vi "Voice_Freq_Amp_Check.vi"(8 "error in (no error)":errorcluster, 11 "IN":T1={"step name 1"="", "updata 2"="750~0.22", "limitdata 3"="650~0.101", "load vi name 4"="", "parameter 5"=""}) -> (0 "error out":errorcluster, 3 "Cluster":T2)   [LabVIEW 2013]
uses:
  <vilib>/sound2/lvsound2.llb/Sampling Mode.ctl
  <vilib>/sound2/lvsound2.llb/Sound Data Format.ctl
  <vilib>/sound2/lvsound2.llb/Sound Input Read (DBL).vi
  <vilib>/measure/matone.llb/Extract Single Tone Information N Chan.vi
  <vilib>/measure/NI_MAPro.lvlib
panel:
  out "array":string[](array[string])
  out "Array":bool[](array[boolean])
  out "number":i32
  # "Hi: 750~0.22"
  # "Lo: 650~0.101"
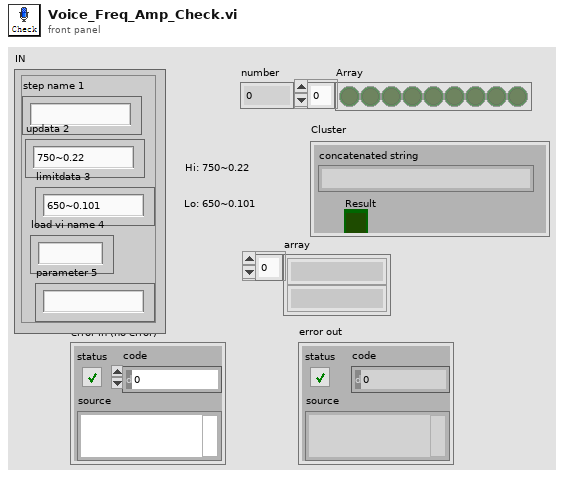
[diagram p1: front panel]
types:
  T1 = cluster{"step name 1":string, "updata 2":string, "limitdata 3":string, "load vi name 4":string, "parameter 5":string}
  T2 = cluster{"concatenated string":string, "Result":bool}
  T3 = typedef "Sound Data Format.ctl" = cluster{"sample rate (S/s)":dbl, "number of channels":i32, "bits per sample":i32}
  T4 = typedef "Sampling Mode.ctl" = i32
  T5 = typedef "Sound Input Task ID.ctl" = u32
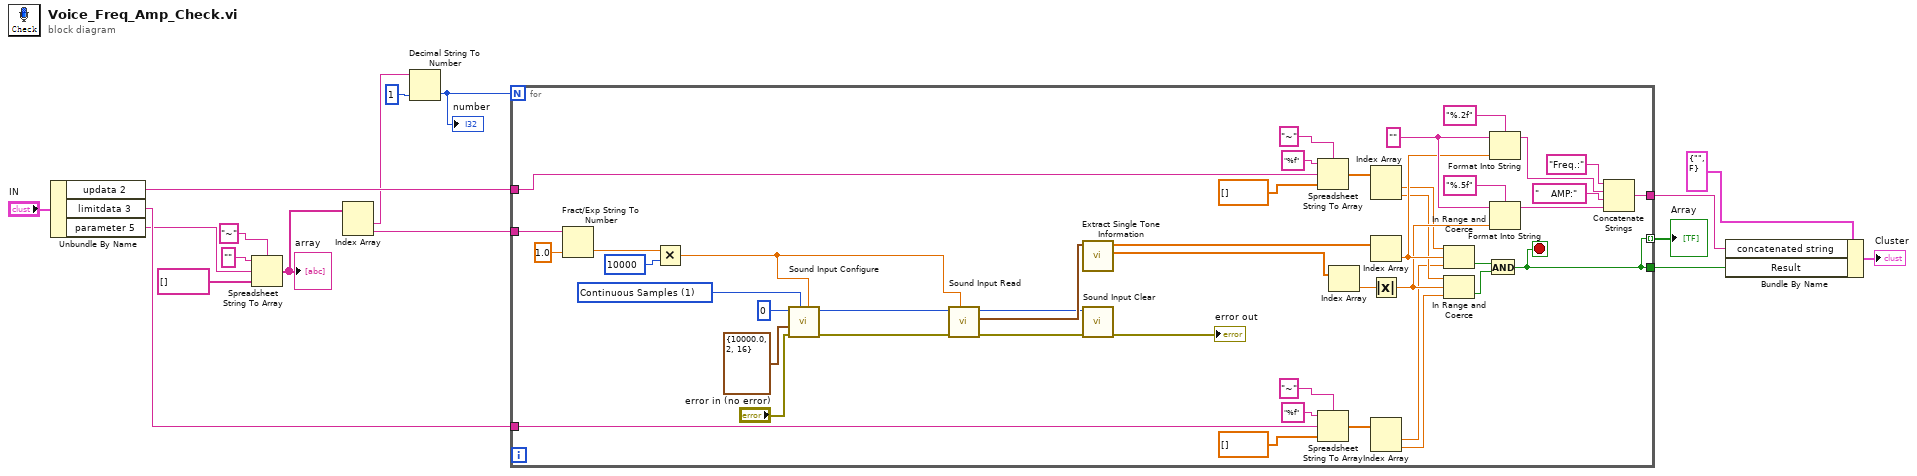
[diagram p0: block diagram]
diagram:
  n1 = Unbundle By Name("IN") -> ("updata 2"=w12:string, "limitdata 3"=w11:string, "parameter 5"=w7:string)
  n2 = Spreadsheet String To Array(delimiter (Tab)="~", format string="", spreadsheet string=w7, array type (2D Dbl)=string[] []) -> (array=w3:string[])
  "array" <- w3
  n3 = Index Array(array=w3) -> (element #1=w2:string, element #2=w1:string)  [unwired: 2 in]
  n4 = Decimal String To Number(string=w2, default (0L)=1 ("default (0 I32)")) -> (number=w9:i32)  [unwired: 1 in, 1 out]
  "number" <- w9
  n5 = for {
    N: w9 -> [_]
    tunnel: [w38] -> w15
    tunnel: [w23] -> w14
    tunnel: w12 -> [w25]
    tunnel: w11 -> [w24]
    tunnel: [w23] -> w8 mode=indexing
    tunnel: w1 -> [w22]
    stop <- w23 stop-if-true
    w49 = "" ("initial string")
    w57 = T4 1 items=["Finite Samples", "Continuous Samples"] ("sample mode")
    n6 = Fract/Exp String To Number(string=w22, default (0 dbl)=1.0 ("default (0 DBL)")) -> (number=w20:dbl)  [unwired: 2 in, 1 out]
    n7 = Multiply(x=w20, y=10000 ("Number of Samples/ch")) -> (x*y=w19:dbl)
    n8 = call <vilib>:"Sound Input Configure.vi"("number of samples/ch"=w19, "sample mode"=w57, "error in (no error)"="error in (no error)", "sound format"=T3 {"sample rate (S/s)"=10000.0, "number of channels"=2, "bits per sample"=16} ("Sound Format"), "device ID"=u32 0 ("Device ID")) -> ("error out"=w52:errorcluster, "task ID"=w54:T5)  [unwired: 2 in, 3 out]
    n9 = call-poly <vilib>:"Sound Input Read.vi"("number of samples/ch"=w19, "error in (no error)"=w52, "task ID"=w54) -> ("error out"=w56:errorcluster, "data"=w61:waveform(dbl)[], "task ID out"=w55:T5)  [unwired: 1 in, 5 out]
    n10 = call-poly <vilib>:"Extract Single Tone Information.vi"("time signals in"=w61) -> ("detected amplitudes"=w60:dbl[], "detected frequencies"=w59:dbl[])  [unwired: 3 in, 6 out]
    n11 = call <vilib>:"Sound Input Clear.vi"("error in (no error)"=w56, "task ID"=w55) -> ("error out"=→"error out":errorcluster)  [unwired: 9 out]
    n12 = Spreadsheet String To Array(delimiter (Tab)="~", format string="%f", spreadsheet string=w25, array type (2D Dbl)=dbl[] []) -> (array=w31:dbl[])
    n13 = Spreadsheet String To Array(delimiter (Tab)="~", format string="%f", spreadsheet string=w24, array type (2D Dbl)=dbl[] []) -> (array=w28:dbl[])
    n14 = Index Array(array=w60) -> (element=w62:dbl)  [unwired: 1 in]
    n15 = Index Array(array=w31) -> (element #1=w30:dbl, element #2=w29:dbl)  [unwired: 2 in]
    n16 = Index Array(array=w59) -> (element=w42:dbl)  [unwired: 1 in]
    n17 = Absolute Value(x=w62) -> (abs(x)=w41:dbl)
    n18 = Index Array(array=w28) -> (element #1=w27:dbl, element #2=w26:dbl)  [unwired: 2 in]
    n19 = In Range and Coerce(upper limit=w30, x=w42, lower limit=w27) -> (In Range?=w40:bool)  [unwired: 1 out]
    n20 = In Range and Coerce(upper limit=w29, x=w41, lower limit=w26) -> (In Range?=w39:bool)  [unwired: 1 out]
    n21 = And(x=w40, y=w39) -> (x .and. y?=w23:bool)
    n22 = Format Into String(format string="%.2f", initial string=w49, w42) -> (resulting string=w47:string)  [unwired: 1 in, 1 out]
    n23 = Format Into String(format string="%.5f", initial string=w49, w41) -> (resulting string=w45:string)  [unwired: 1 in, 1 out]
    n24 = Concatenate Strings("Freq.:" ("string"), w47, "    AMP:" ("string"), w45) -> (w38:string)
  }
  "Array" <- w8
  n25 = Bundle By Name(cluster=T2 {"concatenated string"="", "Result"=FALSE} ("Cluster"), "concatenated string"=w15, "Result"=w14) -> (→"Cluster":T2)
